vi "Get Firmware Program Interfaces.vi"(8 "Error In":errorcluster, 10 "Device ID":u8, 11 "Device Family":T1) -> (0 "Error Out":errorcluster, 3 "Firmware Program Interfaces":string[](array[string]))   [LabVIEW 2013, in "LVH-LINX.lvlib"]
uses:
  <vilib>/LabVIEW Hacker/LINX/LVH-LINX.lvlib
  <vilib>/LabVIEW Hacker/LINX/Private/Type Defs/Device Family.ctl
panel:
  in  "Firmware Program Interface":enum16{"N/A", "Serial / USB", "USB", "TCP"}(ring)
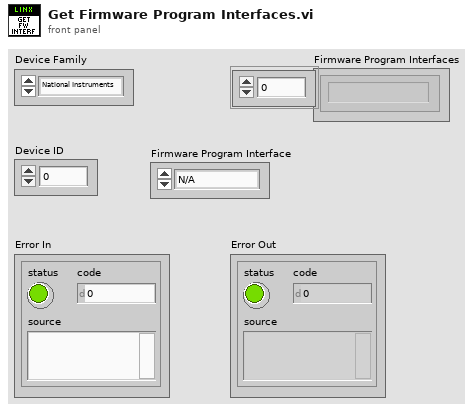
[diagram p1: front panel]
types:
  T1 = typedef "LVH-LINX.lvlib/Device Family.ctl" = enum8{"National Instruments", "Digilent", "Arduino"}
  T2 = typedef "LVH-LINX.lvlib/Generic Device.ctl" = cluster{"DI Channels":u8[], "DO Channels":u8[], "AI":u8[], "AO":u8[], "PWM":u8[], "QE":u8[], "UART":u8[], "I2C 2":u8[], "SPI":u8[], "CAN":u8[], "AI Ref (V)":dbl, "Firmware Program Interfaces":enum16{"N/A", "Serial / USB", "USB", "TCP"}[], "Firmware Versions":T3[], "Name":string, "AO Resolution (Bits)":u8, "AO Ref (V)":dbl}
  T3 = typedef "LVH-LINX.lvlib/Firmware Version.ctl" = cluster{"Name":string, "Relative Path":string, "Firmware Interface":T4}
  T4 = typedef "LVH-LINX.lvlib/Firmware Interface.ctl" = enum32{"Serial ", "Ethernet", "WIFI"}
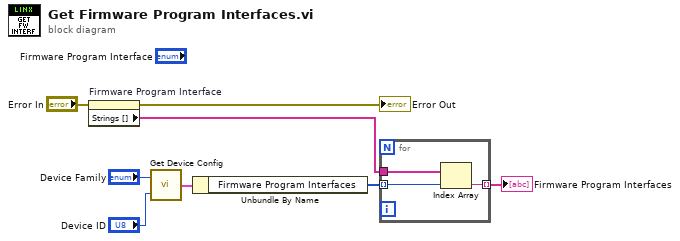
[diagram p0: block diagram]
diagram:
  n1 = property on="Firmware Program Interface" class="Enum (strict)"(error in="Error In") -> (error out=→"Error Out":errorcluster, "Strings []"=w4:string[])  [unwired: 1 in, 1 out]
  n2 = call <vilib>:"Get Device Config.vi"("Device ID"="Device ID", "Device Family"="Device Family") -> ("Device Config"=w7:T2)
  n3 = Unbundle By Name(w7) -> ("Firmware Program Interfaces"=w8:enum16{"N/A", "Serial / USB", "USB", "TCP"}[])
  n4 = for {
    tunnel: w8 -> [w11] mode=indexing
    tunnel: w4 -> [w10]
    tunnel: [w9] -> w3 mode=indexing
    n5 = Index Array(array=w10, index=w11) -> (element=w9:string)
  }
  "Firmware Program Interfaces" <- w3
